vi "Set Row Values.vi"(7 "Sheet Name":string, 8 "error in":errorcluster, 9 "Values":variant[](array[variant]), 10 "Cell Address":string, 11 "SpreadsheetDoc":refnum<k24>) -> (0 "error out":errorcluster, 3 "SpreadsheetDoc out":refnum<k24>)   [LabVIEW 2019, in "Open Xml.lvlib"]
uses:
  Open Xml.lvlib
  D:/git/Open-Xml-LabVIEW/Source/DocumentFormat.OpenXml.dll
  DocumentFormat.OpenXml.dll
  <vilib>/addons/analyzer/_analyzerutils.llb/VIAnUtil Check Type If ErrClust.vi
  <vilib>/Utility/Data Type/NI_Data Type.lvlib
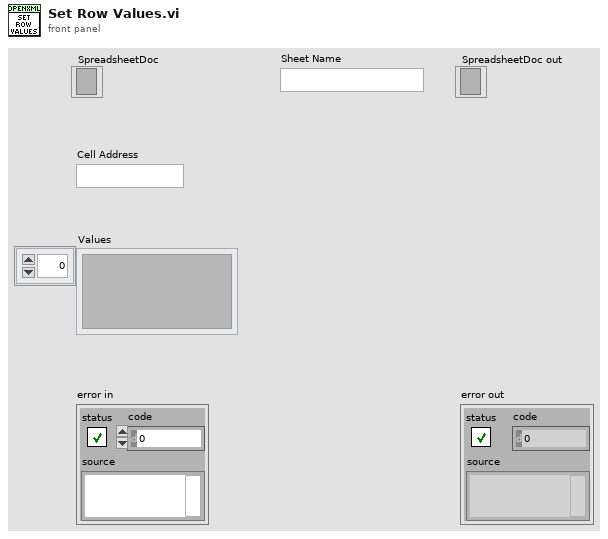
[diagram p1: front panel]
types:
  T1 = typedef "NI_Data Type.lvlib/Data Type.ctl" = enum8{"Invalid Type", "Void", "I8", "I16", "I32", "I64", "U8", "U16", "U32", "U64", "Single Float", "Double Float", "Extended Float", "Single Complex", "Double Complex", "Extended Complex", "Enum U8", "Enum U16", "Enum U32", "Enum U64", "Single Float With Unit", "Double Float With Unit", "Extended Float With Unit", "Single Complex with Unit", "Double Complex with Unit", "Extended Complex with Unit", "Boolean", "String", "Path", "Picture", "Tag", "Array", "Cluster", "Variant", "LV Variant", "Waveform", "Timestamp", "Digital Waveform", "Digital Data", "ExpressData", "Refnum", "External Data", "VI", "Poly VI", "LabVIEW Class Instance", "Fixed Point", "Set Collection", "Map Collection"}
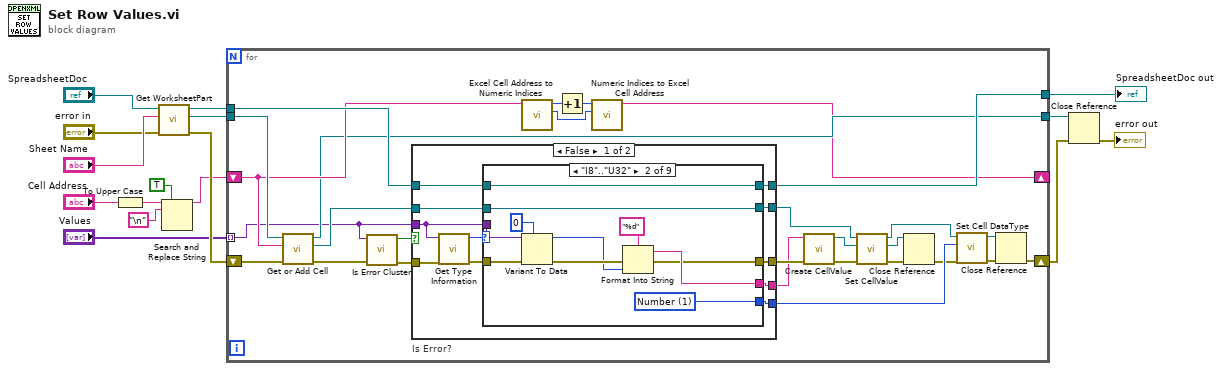
[diagram p0: block diagram]
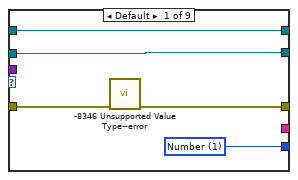
[diagram p2: hidden frame]
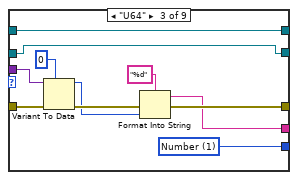
[diagram p3: hidden frame]
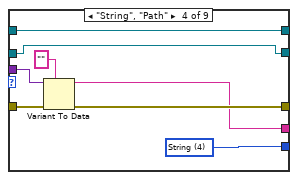
[diagram p4: hidden frame]
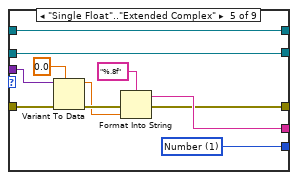
[diagram p5: hidden frame]
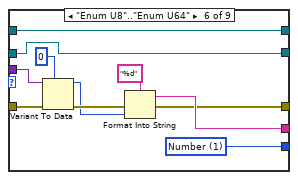
[diagram p6: hidden frame]
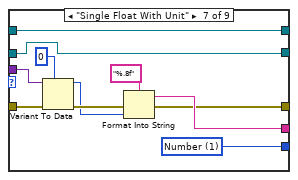
[diagram p7: hidden frame]
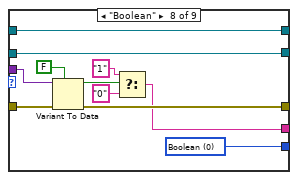
[diagram p8: hidden frame]
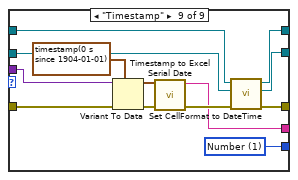
[diagram p9: hidden frame]
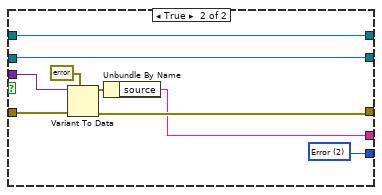
[diagram p10: hidden frame]
diagram:
  n1 = To Upper Case(1:"Cell Address") -> (0:w4:string)
  n2 = call "Get WorksheetPart.vi"("error in"="error in", "Sheet Name"="Sheet Name", "SpreadsheetDocument in"="SpreadsheetDoc") -> ("error out"=w14:errorcluster, "WorksheetPart"=w13:refnum<k24>, "SpreadsheetDocument out"=w11:refnum<k24>)  [unwired: 6 in]
  n3 = Search and Replace String(replace all?=TRUE ("replace all? (F)"), input string=w4, search string="\n") -> (result string=w3:string)  [unwired: 5 in, 3 out]
  n4 = for {
    tunnel: "Values" -> [w19] mode=indexing
    shift-right: [w34] -> w15
    shift-left: w14 -> [w44]
    shift-right: [w22] -> _
    shift-left: w3 -> [w24]
    tunnel: w13 -> [w31]
    tunnel: w11 -> [w29]
    tunnel: [w28] -> w9
    tunnel: [w23] -> w1
    n5 = call "Get or Add Cell.vi"("error in"=w44, "Cell Address"=w24, "Worksheetpart in"=w31) -> ("error out"=w21:errorcluster, "Cell"=w30:refnum<k24>, "WorksheetPart out"=w23:refnum<k24>)  [unwired: 6 in]
    n6 = call <vilib>:"Is Error Cluster.vi"("error in (no error)"=w21, "variant"=w19) -> ("error out"=w20:errorcluster, "is error cluster?"=w18:bool)  [unwired: 8 in]
    n7 = case "Is Error?" shown="False" w18 {
      tunnel: [w53 w152] -> w41
      tunnel: [w52 w149] -> w39
      tunnel: [w51 w151] -> w32
      tunnel: w30 -> [w50 w148]
      tunnel: w29 -> [w49 w147]
      tunnel: [w48 w147] -> w28
      tunnel: [w47 w148] -> w27
      tunnel: w20 -> [w46 w155]
      tunnel: w19 -> [w45 w153]
      frame False {
        n8 = call <vilib>:"Get Type Information.vi"("error in (no error)"=w46, "variant"=w45) -> ("error out"=w55:errorcluster, "type"=w54:T1)  [unwired: 5 in, 3 out]
        n9 = case shown="\"I8\"..\"U32\"" w54 {
          tunnel: w55 -> [w60 w71 w82 w90 w101 w112 w123 w134 w146]
          tunnel: w45 -> [_ w67 w80 w88 w96 w107 w118 w133 w144]
          tunnel: [_ w69 w75 w86 w99 w110 w121 w127 w141] -> w52
          tunnel: [w59 w64 w78 w87 w98 w109 w120 w131 w139] -> w53
          tunnel: [w58 w63 w74 w85 w93 w104 w116 w126 w140] -> w51
          tunnel: w50 -> [w57 w62 w72 w83 w91 w102 w113 w124 w138]
          tunnel: w49 -> [w56 w61 w73 w84 w92 w103 w114 w125 w137]
          tunnel: [w56 w61 w73 w84 w92 w103 w114 w125 w136] -> w48
          tunnel: [w57 w62 w72 w83 w91 w102 w113 w124 w135] -> w47
          frame Default {
            w58 = 1 items=["Boolean", "Number", "Error", "SharedString", "String", "InlineString", "Date"] ("Datatype")
            n10 = call "-8346 Unsupported Value Type--error.vi"("error in"=w60) -> ("error out"=w59:errorcluster)  [unwired: 10 in]
          }
          frame "I8".."U32" {
            w63 = 1 items=["Boolean", "Number", "Error", "SharedString", "String", "InlineString", "Date"] ("Datatype")
            n11 = Variant To Data(error in=w71, type=i64 0, Variant=w67) -> (data=w65:i64, error out=w68:errorcluster)
            n12 = Format Into String(format string="%d", error in=w68, w65) -> (resulting string=w69:string, error out=w64:errorcluster)  [unwired: 1 in]
          }
          frame "U64" {
            w74 = 1 items=["Boolean", "Number", "Error", "SharedString", "String", "InlineString", "Date"] ("Datatype")
            n13 = Variant To Data(error in=w82, type=u64 0, Variant=w80) -> (data=w77:u64, error out=w79:errorcluster)
            n14 = Format Into String(format string="%d", error in=w79, w77) -> (resulting string=w75:string, error out=w78:errorcluster)  [unwired: 1 in]
          }
          frame "String", "Path" {
            w85 = 4 items=["Boolean", "Number", "Error", "SharedString", "String", "InlineString", "Date"] ("Datatype")
            n15 = Variant To Data(error in=w90, type="", Variant=w88) -> (data=w86:string, error out=w87:errorcluster)
          }
          frame "Single Float".."Extended Complex" {
            w93 = 1 items=["Boolean", "Number", "Error", "SharedString", "String", "InlineString", "Date"] ("Datatype")
            n16 = Variant To Data(error in=w101, type=0.0, Variant=w96) -> (data=w94:dbl, error out=w97:errorcluster)
            n17 = Format Into String(format string="%.8f", error in=w97, w94) -> (resulting string=w99:string, error out=w98:errorcluster)  [unwired: 1 in]
          }
          frame "Enum U8".."Enum U64" {
            w104 = 1 items=["Boolean", "Number", "Error", "SharedString", "String", "InlineString", "Date"] ("Datatype")
            n18 = Variant To Data(error in=w112, type=u64 0, Variant=w107) -> (data=w105:u64, error out=w108:errorcluster)
            n19 = Format Into String(format string="%d", error in=w108, w105) -> (resulting string=w110:string, error out=w109:errorcluster)  [unwired: 1 in]
          }
          frame "Single Float With Unit" {
            w116 = 1 items=["Boolean", "Number", "Error", "SharedString", "String", "InlineString", "Date"] ("Datatype")
            n20 = Variant To Data(error in=w123, type=u64 0, Variant=w118) -> (data=w115:u64, error out=w119:errorcluster)
            n21 = Format Into String(format string="%.8f", error in=w119, w115) -> (resulting string=w121:string, error out=w120:errorcluster)  [unwired: 1 in]
          }
          frame "Boolean" {
            w126 = 0 items=["Boolean", "Number", "Error", "SharedString", "String", "InlineString", "Date"] ("Datatype")
            n22 = Variant To Data(error in=w134, type=FALSE, Variant=w133) -> (data=w130:bool, error out=w131:errorcluster)
            n23 = Select(t="1", s=w130, f="0") -> (s? t:f=w127:string)
          }
          frame "Timestamp" {
            w140 = 1 items=["Boolean", "Number", "Error", "SharedString", "String", "InlineString", "Date"] ("Datatype")
            n24 = Variant To Data(error in=w146, type=timestamp(0 s since 1904-01-01), Variant=w144) -> (data=w143:timestamp, error out=w145:errorcluster)
            n25 = call "Timestamp to Excel Serial Date.vi"("Timestamp"=w143) -> ("Excel Serial Date"=w141:string)  [unwired: 10 in]
            n26 = call "Set CellFormat to DateTime.vi"("error in"=w145, "Cell in"=w138, "SpreadsheetDoc in"=w137) -> ("error out"=w139:errorcluster, "Cell out"=w135:refnum<k24>, "SpreadsheetDocument out"=w136:refnum<k24>)  [unwired: 6 in]
          }
        }
      }
      frame True {
        w151 = 2 items=["Boolean", "Number", "Error", "SharedString", "String", "InlineString", "Date"] ("Datatype")
        n27 = Variant To Data(error in=w155, type=errorcluster {"status"=FALSE, "code"=0, "source"=""} ("error constant"), Variant=w153) -> (data=w150:errorcluster, error out=w152:errorcluster)
        n28 = Unbundle By Name(w150) -> ("source"=w149:string)
      }
    }
    n29 = call "Excel Cell Address to Numeric Indices.vi"("Cell Name"=w24) -> ("Row Number"=w17:i32, "Column Number"=w43:i32)  [unwired: 9 in]
    n30 = Increment(x=w43) -> (x+1=w42:i32)
    n31 = call "Numeric Indices to Excel Cell Address.vi"("Row"=w17, "Column"=w42) -> ("Cell Address"=w22:string)  [unwired: 9 in]
    n32 = call "Create CellValue.vi"("error in"=w41, "Text"=w39) -> ("error out"=w40:errorcluster, "CellValue out"=w37:refnum<k24>)  [unwired: 8 in]
    n33 = call "Set CellValue.vi"("error in"=w40, "CellValue in"=w37, "Cell in"=w27) -> ("error out"=w38:errorcluster, "CellValue out"=w26:refnum<k24>, "Cell out"=w35:refnum<k24>)  [unwired: 6 in]
    n34 = Close Reference(reference=w26, error in (no error)=w38) -> (error out=w25:errorcluster)
    n35 = call "Set Cell DataType.vi"("error in"=w25, "Datatype"=w32, "Cell in"=w35) -> ("error out"=w36:errorcluster, "Cell out"=w33:refnum<k24>)  [unwired: 7 in]
    n36 = Close Reference(reference=w33, error in (no error)=w36) -> (error out=w34:errorcluster)
  }
  "SpreadsheetDoc out" <- w9
  n37 = Close Reference(reference=w1, error in (no error)=w15) -> (error out=→"error out":errorcluster)
